vi "RS_RTO1024_FASTQUERY.vi"(7 "input":string, 8 "error in":T6, 11 "DriverConnect in":T1={"InterfaceType"=enum."VISA", "OpenedSession"="", "InterfaceSettings"={"Interface"=enum."RS232", "EOS 4 read"=enum."LF (\\n)", "EOS 4 write"=enum."LF (\\n)", "TMO, ms"=10000, "Sett"=variant(cluster{"Baud Rate":u32, "Data Bits":u16, "Parity":u16, "Stop Bits":u16, "Flow Control":u16, "Eho":bool} {"Baud Rate"=75, "Data Bits"=0, "Parity"=0, "Stop Bits"=0, "Flow Control"=0, "Eho"=FALSE})}}) -> (0 "error out":T6, 3 "DriverConnect out":T1={"InterfaceType"=enum."VISA", "OpenedSession"="", "InterfaceSettings"={"Interface"=enum."RS232", "EOS 4 read"=enum."LF (\\n)", "EOS 4 write"=enum."LF (\\n)", "TMO, ms"=10000, "Sett"=variant(cluster{"Baud Rate":u32, "Data Bits":u16, "Parity":u16, "Stop Bits":u16, "Flow Control":u16, "Eho":bool} {"Baud Rate"=75, "Data Bits"=0, "Parity"=0, "Stop Bits"=0, "Flow Control"=0, "Eho"=FALSE})}}, 4 "output":string)   [LabVIEW 2018]
uses:
  MOKO_LabViewLibrary/MokoLowLevel/MokoLowLovelControl/MLLC_Error.ctl
  MOKO_LabViewLibrary/MokoLowLevel/MokoLowLovelControl/MLLC_ConnectCluster.ctl
  MOKO_LabViewLibrary/MokoLowLevel/MokoLowLovelControl/MLLC_InterfaceType.ctl
  MOKO_LabViewLibrary/MokoLowLevel/MokoLowLovelControl/MLLC_OpenedSession.ctl
  MOKO_LabViewLibrary/MokoLowLevel/MokoLowLovelControl/MLLC_InterfaceSettings.ctl
  MOKO_LabViewLibrary/MokoLowLevel/MokoLowLovelControl/MLLC_InterfaceKind.ctl
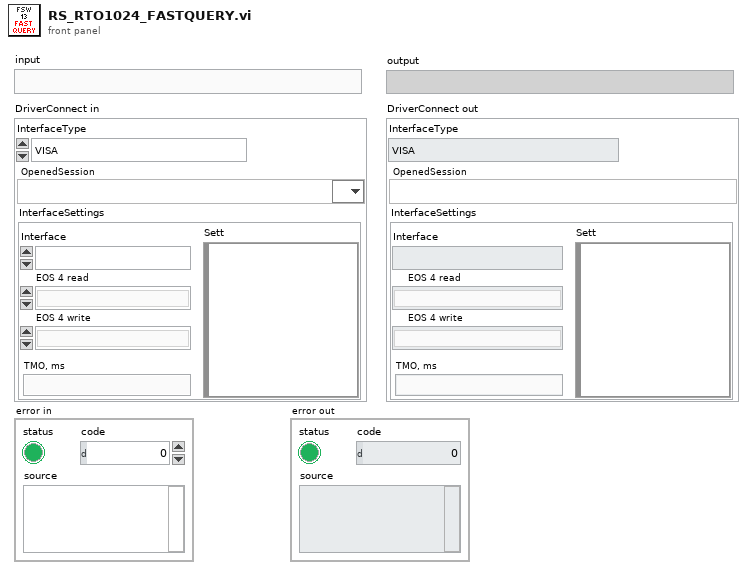
[diagram p1: front panel]
types:
  T1 = typedef "MLLC_ConnectCluster.ctl" = cluster{"InterfaceType":T2, "OpenedSession":T3, "InterfaceSettings":T4}
  T2 = typedef "MLLC_InterfaceType.ctl" = enum16{"VISA", "Prologix USB-GPIB"}
  T3 = typedef "MLLC_OpenedSession.ctl" = refnum<visa-resource-name>
  T4 = typedef "MLLC_InterfaceSettings.ctl" = cluster{"Interface":T5, "EOS 4 read":enum16{"Default (=EOS 4 write)", "CR (\\r)", "LF (\\n)", "None"}, "EOS 4 write":enum16{"CR+LF (\\r\\n)", "CR (\\r)", "LF (\\n)", "None"}, "TMO, ms":i32, "Sett":variant}
  T5 = typedef "MLLC_InterfaceKind.ctl" = enum16{"RS232", "GPIB", "USB", "Ethernet", "another"}
  T6 = typedef "MLLC_Error.ctl" = errorcluster
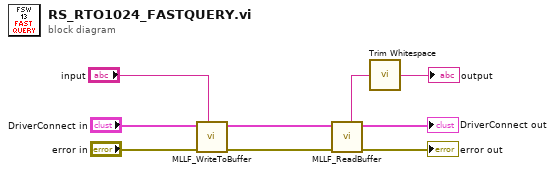
[diagram p0: block diagram]
diagram:
  n1 = call "MLLF_WriteToBuffer.vi"("String"="input", "error in"="error in", "DriverConnect in"="DriverConnect in") -> ("error out"=w3:T6, "DriverConnect out"=w4:T1)  [unwired: 5 in]
  n2 = call "MLLF_ReadBuffer.vi"("Error In"=w3, "DriverConnect in"=w4) -> ("Error Out"=→"error out":errorcluster, "DriverConnect out"=→"DriverConnect out":T1, "String"=w5:string)  [unwired: 6 in]
  n3 = call <vilib>:"Trim Whitespace.vi"("string"=w5) -> ("trimmed string"=→"output":string)  [unwired: 1 in]
